vi "FittingForAutofocus.vi"(9 "Step size":dbl, 11 "Differences":dbl[](array[numeric])) -> (0 "fit coefficnets":dbl[](array[numeric]), 1 "Outside range":bool, 3 "Move by":dbl)   [LabVIEW 2015]
uses:
  <vilib>/imath/engines/lvmath2/RunTimeEngine/Managers/WorkSpace/UID Generator.vi
  <vilib>/imath/engines/lvmath2/RunTimeEngine/RunTimeType/NIMS_RunTimeType_From StrictType (excl LVString).vi
  <instcachedir>/0/NIMS_RunTimeType_From StrictType (excl LVString)_EB1C38A9BC5048DA9ABDA8F781E54D21.lvgen/NIMS_RunTimeType_From StrictType (excl LVString)_EB1C38A9BC5048DA9ABDA8F781E54D21_000.vi
  <vilib>/imath/engines/lvmath2/RunTimeEngine/LocalVariableDefStatement/MC_LocalVariableDefStatement_Display.vi
  <vilib>/imath/engines/lvmath2/RunTimeEngine/ArithmeticOperatorToken/NIMS_ArithmeticOperator_power(S).vi
  <instcachedir>/0/NIMS_ArithmeticOperator_power(S)_DFB67823F1414E5097C86E39787D8CA8.lvgen/NIMS_ArithmeticOperator_power(S)_DFB67823F1414E5097C86E39787D8CA8_010.vi
  <vilib>/imath/engines/lvmath2/RunTimeEngine/ErrorHandling/NIMS_Create Error From Enums.vi
  <vilib>/imath/engines/lvmath2/RunTimeEngine/BuiltInFunctions/double/NIMS_double.vi
  <instcachedir>/0/NIMS_double_34E32F64C2B04A25A042F4CA881A0A41.lvgen/NIMS_double_34E32F64C2B04A25A042F4CA881A0A41_002.vi
  <vilib>/imath/engines/lvmath2/RunTimeEngine/Managers/SymbolTable/Clear UID.vi
  <vilib>/imath/engines/lvmath2/RunTimeEngine/NodeEndStatement/NIMS_NodeEndStatement_Output.vi
  <instcachedir>/0/NIMS_NodeEndStatement_Output_53EC0D466D134D7ABD903AC30B43404B.lvgen/NIMS_NodeEndStatement_Output_53EC0D466D134D7ABD903AC30B43404B_009.vi
  <vilib>/imath/engines/lvmath2/RunTimeEngine/ErrorHandling/NIMS_Finalize Error.vi
  <vilib>/Analysis/NI_AALPro.lvlib
  <vilib>/imath/engines/lvmath2/RunTimeEngine/Managers/SymbolTable/NIMS_WorkSpace.lvlib
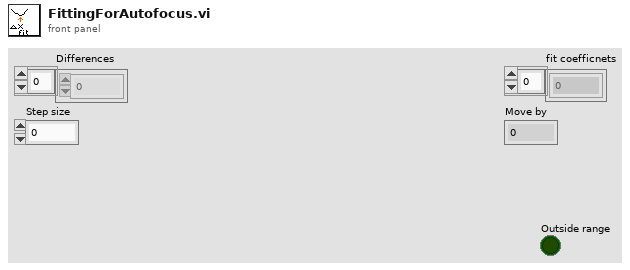
[diagram p1: front panel]
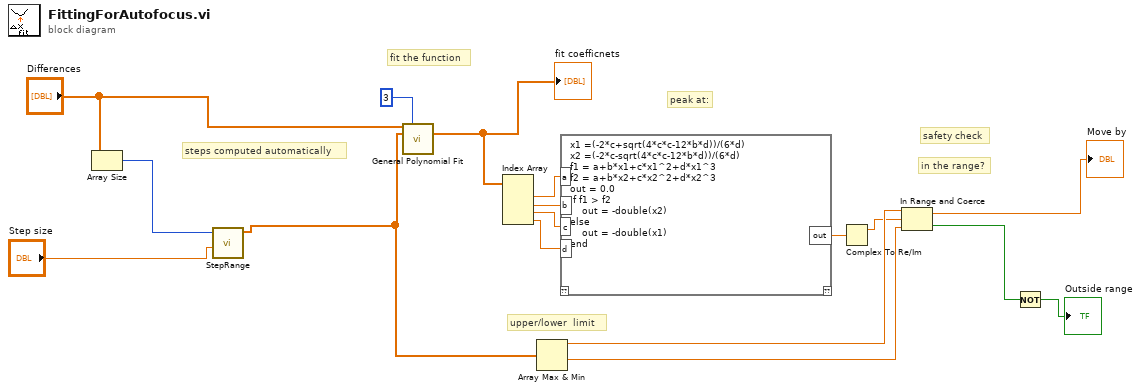
[diagram p0: block diagram]
diagram:
  # "upper/lower  limit"
  # "in the range?"
  # "safety check"
  # "peak at:"
  # "fit the function"
  # "steps computed automatically"
  n1 = Array Size(array="Differences") -> (size(s)=w9:i32)
  n2 = call "StepRange.vi"("Step size (um)"="Step size", "Number of Steps"=w9) -> ("Displacements (um)"=w7:dbl[])  [unwired: 8 in, 1 out]
  n3 = call <vilib>:"General Polynomial Fit.vi"("Y"="Differences", "polynomial order"=3, "X"=w7) -> ("Polynomial Coefficients"=w15:dbl[])  [unwired: 9 in, 3 out]
  "fit coefficnets" <- w15
  n4 = Index Array(array=w15) -> (element #1=w6:dbl, element #2=w5:dbl, element #3=w4:dbl, element #4=w3:dbl)  [unwired: 4 in]
  n5 = Array Max & Min(array=w7) -> (max value=w13:dbl, min value=w12:dbl)  [unwired: 2 out]
  n6 = mathscript code="x1 =(-2*c+sqrt(4*c*c-12*b*d))/(6*d) \nx2 =(-2*c-sqrt(4*c*c-12*b*d))/(6*d) \nf1 = a+b*x1+c*x1^2+d*x1^3\nf2 = a+b*x2+c*x2^2+d*x2^3\nout = 0.0\nif f1 > f2\n    out = -double(x2)\nelse \n    out = -double(x1)\nend"("a"=w6, "b"=w5, "c"=w4, "d"=w3) -> ("out"=w2:cdb)  [unwired: 1 in, 1 out]
  n7 = Complex To Re/Im(x + iy=w2) -> (x=w1:dbl)  [unwired: 1 out]
  n8 = In Range and Coerce(upper limit=w13, x=w1, lower limit=w12) -> (coerced(x)=→"Move by":dbl, In Range?=w10:bool)
  n9 = Not(x=w10) -> (.not. x?=→"Outside range":bool)
